vi "create encoder edge direction command.vi"(10 "Falling edge?":bool=TRUE) -> (3 "command message":variant)   [LabVIEW 2018]
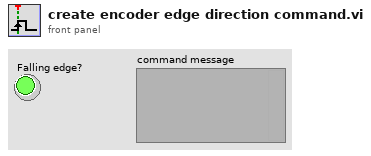
[diagram p1: front panel]
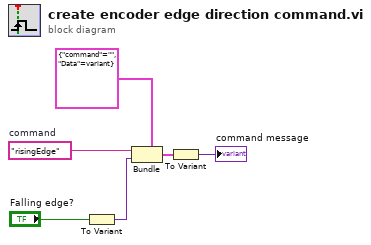
[diagram p0: block diagram]
diagram:
  w5 = "risingEdge"  # command
  n1 = To Variant(anything="Falling edge?") -> (Variant=w4:variant)
  n2 = Bundle(cluster=cluster{"command":string, "Data":variant} {"command"="", "Data"=variant}, "command"=w5, "Data"=w4) -> (w3:cluster{"command":string, "Data":variant})
  n3 = To Variant(anything=w3) -> (Variant=→"command message":variant)
